vi "SLSC Search Item in Tree Control.vi"(0 "SLSC Output Tree":T1(array[cluster]), 5 "Item Tag":string) -> (4 "SLSC Output Tree Out":T1(array[cluster]), 6 "Found?":bool, 8 "Position":i32, 10 "Item":T2)   [LabVIEW 2017, in "SLSC Tree Control.lvlib"]
doc: "Searches for a specific item tag in the SLSC Output Tree."
uses:
  SLSC Tree Control.lvlib
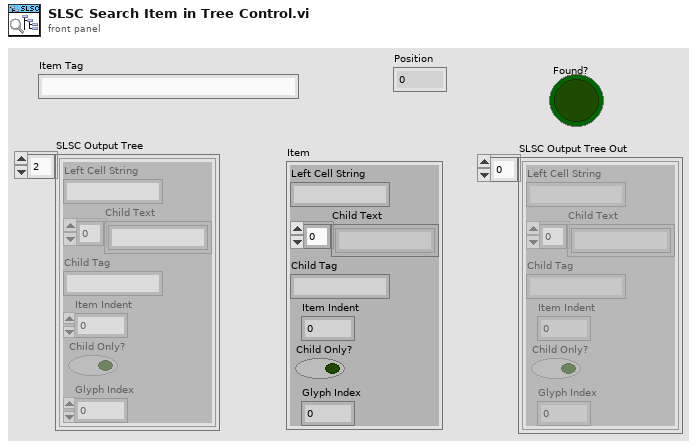
[diagram p1: front panel]
types:
  T1 = cluster{"Left Cell String":string, "Child Text":string[], "Child Tag":string, "Item Indent":i32, "Child Only?":bool, "Glyph Index":i32}[]
  T2 = cluster{"Left Cell String":string, "Child Text":string[], "Child Tag":string, "Item Indent":i32, "Child Only?":bool, "Glyph Index":i32}
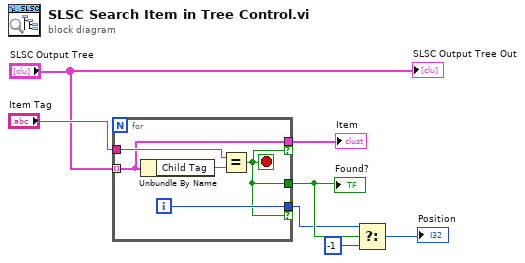
[diagram p0: block diagram]
diagram:
  n1 = for {
    tunnel: "SLSC Output Tree" -> [w10] mode=indexing
    tunnel: "Item Tag" -> [w11]
    tunnel: [w10] -> w7 if=w8
    tunnel: [w8] -> w4
    tunnel: [w9] -> w3 if=w8
    i -> [w9]
    stop <- w8 stop-if-true
    n2 = Unbundle By Name(w10) -> ("Child Tag"=w12:string)
    n3 = Equal?(x=w11, y=w12) -> (x = y?=w8:bool)
  }
  "Item" <- w7
  "Found?" <- w4
  n4 = Select(t=w3, s=w4, f=-1) -> (s? t:f=→"Position":i32)
  "SLSC Output Tree Out" <- "SLSC Output Tree"
